vi "create dispatcher.vi"(8 "error in":errorcluster, 11 "pool sizes (standard=10)":T1={"UI thread"=0, "standard"=10, "instrument I/O"=0, "data acquisition"=0, "other 1"=0, "other 2"=0}) -> (0 "error out":errorcluster, 3 "dispatcher":refnum<class "thread pool.lvclass">)   [LabVIEW 2015, in "thread pool.lvclass"]
uses:
  thread pool.lvclass
  pool sizes.ctl
  thread pool.lvclass/thread pool.ctl
  results reporter/results reporter.lvclass
  task/task.lvclass
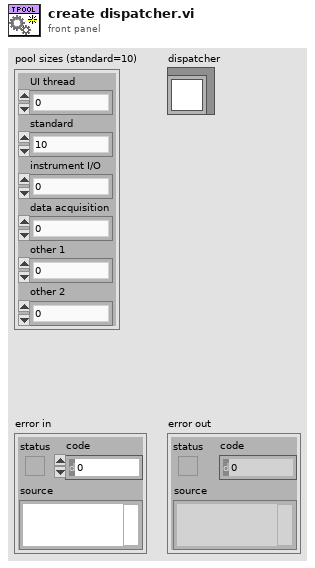
[diagram p1: front panel]
types:
  T1 = typedef "thread pool.lvclass/pool sizes.ctl" = cluster{"UI thread":u8, "standard":u8, "instrument I/O":u8, "data acquisition":u8, "other 1":u8, "other 2":u8}
  T2 = typedef "thread pool.lvclass/vi references.ctl" = cluster{"UI thread":T3, "standard":T3, "instrument I/O":T3, "data acquisition":T3, "other 1":T3, "other 2":T3}
  T3 = typedef "thread pool.lvclass/strict executor reference.ctl" = refnum<vi>
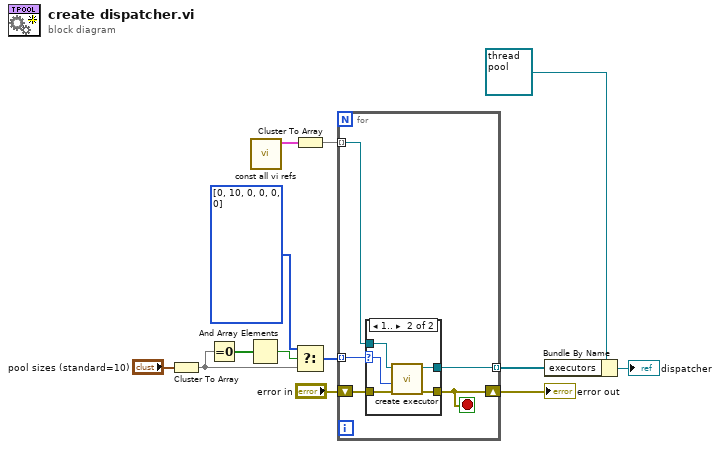
[diagram p0: block diagram]
diagram:
  n1 = Cluster To Array(cluster="pool sizes (standard=10)") -> (array=w9:u8[])
  n2 = Equal To 0?(x=w9) -> (x = 0?=w12:bool[])
  n3 = And Array Elements(Boolean array=w12) -> (logical AND=w11:bool)
  n4 = call "const all vi refs.vi"() -> ("initial pool sizes"=w3:T2)  [unwired: 11 in]
  n5 = Cluster To Array(cluster=w3) -> (array=w2:T3[])
  n6 = Select(t=u8[] [0, 10, 0, 0, 0, 0] ("array"), s=w11, f=w9) -> (s? t:f=w7:u8[])
  n7 = for {
    tunnel: w7 -> [w14] mode=indexing
    tunnel: [w18] -> w6 mode=indexing
    shift-right: [w16] -> w4
    shift-left: "error in" -> [w17]
    tunnel: w2 -> [w15] mode=indexing
    stop <- w16 stop-if-true
    n8 = case shown="1.." w14 {
      selector: w14 -> [_ w20]
      tunnel: [_ w24] -> w18
      tunnel: w17 -> [w19 w23]
      tunnel: [w19 w22] -> w16
      tunnel: w15 -> [_ w21]
      frame ..0 {
      }
      frame 1.. {
        n9 = call "create executor.vi"("error in"=w23, "default pool size"=w20, "launcher ref"=w21) -> ("error out"=w22:errorcluster, "executor reference"=w24:T3)  [unwired: 7 in]
      }
    }
  }
  "error out" <- w4
  n10 = Bundle By Name(cluster=refnum<class "thread pool.lvclass"> refnum ("dispatcher.lvclass"), "executors"=w6) -> (→"dispatcher":refnum<class "thread pool.lvclass">)
